vi "Enumerate Chassis.vi"(8 "error in (no error)":errorcluster) -> (0 "error out":errorcluster, 3 "Chassis":T1[](array[typedef]))   [LabVIEW 2019, in "DAQmx.lvclass"]
uses:
  DAQmx.lvclass
  typedefs/DeviceInfo--Cluster.ctl
  <vilib>/nisyscfg/Filter Mode.ctl
  <vilib>/nisyscfg/Close (Filter).vi
  <vilib>/nisyscfg/Close (Hardware).vi
  <vilib>/nisyscfg/Close (System).vi
  <resource>/objmgr/nicontrollersysapi.rc
  <vilib>/nisyscfg/nisyscfg.lvlib
  <resource>/objmgr/nisysapi.rc
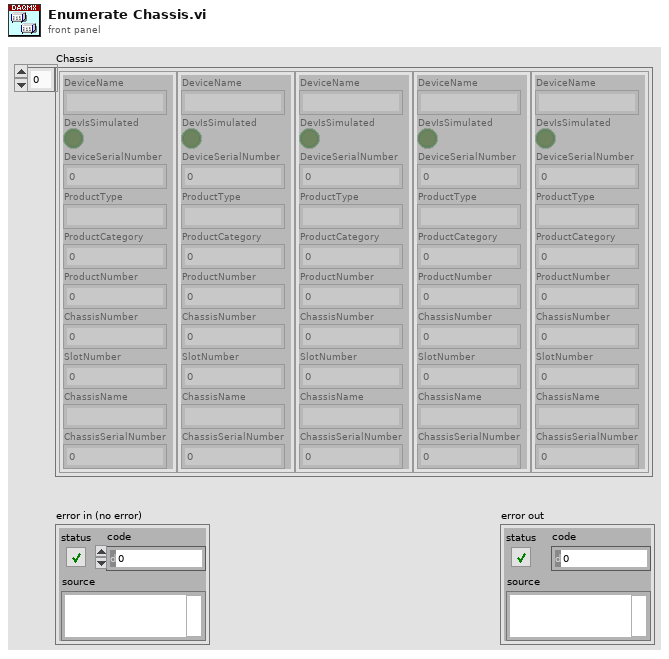
[diagram p1: front panel]
types:
  T1 = typedef "DAQmx.lvclass/DeviceInfo--Cluster.ctl" = cluster{"DeviceName":string, "DevIsSimulated":bool, "DeviceSerialNumber":u32, "ProductType":string, "ProductCategory":i32, "ProductNumber":u32, "ChassisNumber":u32, "SlotNumber":u32, "ChassisName":string, "ChassisSerialNumber":u32}
  T2 = typedef "nisyscfg.lvlib/Filter Mode.ctl" = i32
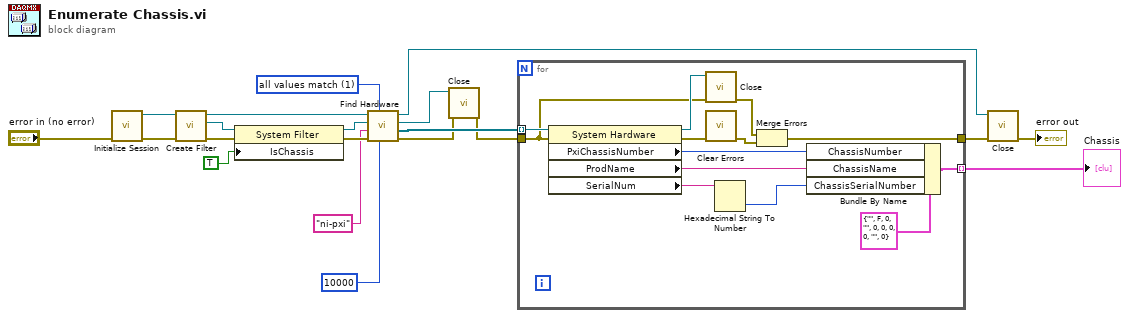
[diagram p0: block diagram]
diagram:
  w9 = T2 1 items=["all values match"=1, "any value matches"=2, "values do not match"=3, "all properties exist"=4] ("Filter Mode (all values match)")
  n1 = call <vilib>:"Initialize Session.vi"("error in (no error)"="error in (no error)") -> ("error out"=w6:errorcluster, "Session out"=w8:refnum<k21>)  [unwired: 9 in]
  n2 = call <vilib>:"Create Filter.vi"("error in (no error)"=w6, "Session in"=w8) -> ("error out"=w17:errorcluster, "Filter out"=w16:refnum<k20>, "Session out"=w15:refnum<k21>)  [unwired: 7 in]
  n3 = property class="System Filter"(reference=w16, error in=w17, "IsChassis"=TRUE ("Is Chassis")) -> (reference out=w14:refnum<k20>, error out=w13:errorcluster)
  n4 = call <vilib>:"Find Hardware.vi"("Remote Timeout (300,000 ms)"=u32 10000, "Filter Mode (all values match)"=w9, "error in (no error)"=w13, "Experts"="ni-pxi", "Filter in"=w14, "Session in"=w15) -> ("error out"=w2:errorcluster, "Resources out"=w19:refnum<k20>[], "Filter out"=w3:refnum<k20>, "Session out"=w5:refnum<k21>)  [unwired: 2 in]
  n5 = call-poly <vilib>:"Close.vi"("error in (no error)"=w2, "Filter in"=w3) -> ("error out"=w1:errorcluster)  [unwired: 9 in]
  n6 = for {
    tunnel: w19 -> [w33] mode=indexing
    tunnel: w1 -> [w28]
    tunnel: [w31] -> w18
    tunnel: [w23] -> w4 mode=indexing
    n7 = property class="System Hardware"(reference=w33, error in=w28) -> (reference out=w32:refnum<k20>, error out=w30:errorcluster, "PxiChassisNumber"=w26:u32, "ProdName"=w25:string, "SerialNum"=w22:string)
    n8 = call-poly <vilib>:"Close.vi"("error in (no error)"=w28, "Resource in"=w32) -> ("error out"=w29:errorcluster)  [unwired: 9 in]
    n9 = call <vilib>:"Clear Errors.vi"("error in (no error)"=w30) -> ("error out"=w27:errorcluster)  [unwired: 5 in, 1 out]
    n10 = Hexadecimal String To Number(string=w22) -> (number=w21:u32)  [unwired: 2 in, 1 out]
    n11 = Merge Errors(w29, w27) -> (w31:errorcluster)
    n12 = Bundle By Name(cluster=T1 {"DeviceName"="", "DevIsSimulated"=FALSE, "DeviceSerialNumber"=0, "ProductType"="", "ProductCategory"=0, "ProductNumber"=0, "ChassisNumber"=0, "SlotNumber"=0, "ChassisName"="", "ChassisSerialNumber"=0} ("Device"), "ChassisNumber"=w26, "ChassisName"=w25, "ChassisSerialNumber"=w21) -> (w23:T1)
  }
  "Chassis" <- w4
  n13 = call-poly <vilib>:"Close.vi"("error in (no error)"=w18, "Session in"=w5) -> ("error out"=→"error out":errorcluster)  [unwired: 9 in]
